vi "UpdateWeightsOutputLayer.vi"(0 "OutputH2":sgl[](array[numeric])=[0.0, 0.0], 1 "Final Output":sgl, 3 "dEtot_dOut":sgl, 4 "Learning Rate":sgl) -> ()   [LabVIEW 2020]
uses:
  <vilib>/rvi/Emulation/niFpgaSctlEmulationGetInTimedLoop.vi
  Global var FPGA.vi
  <vilib>/rvi/Memory/Memory_Emulation/nirvimemoryFastEmulation.vi
  <vilib>/rvi/Memory/Memory_Emulation/nirvimemoryEmulation.vi
  <vilib>/rvi/Emulation/niFpgaEmulationIsFPGAContextNoSignature.vi
  <vilib>/rvi/DataTransferAndStorage/Container/Common/niFpgaContainerGetUniqueNameForEmu.vi
  <vilib>/rvi/Emulation/niFpgaProcessEmulError.vi
  <vilib>/rvi/errors/nirviReportUnexpectedCaseInternalError (U32).vi
  <vilib>/rvi/DataTransferAndStorage/Container/XNode/niFpgaContainer.xnode
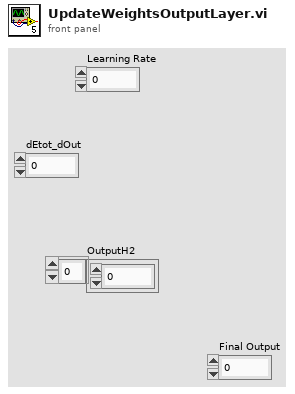
[diagram p1: front panel]
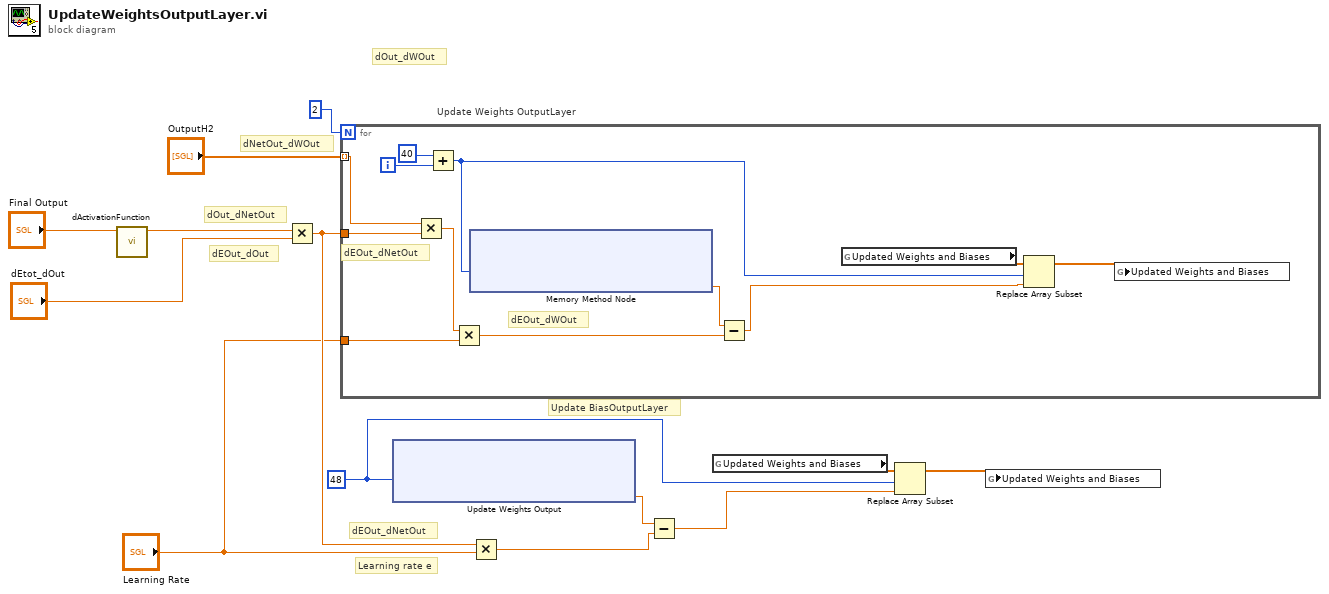
[diagram p0: block diagram]
diagram:
  w3 = u32 48 ("Address")
  # "Learning rate e"
  # "dEOut_dNetOut"
  # "dOut_dWOut"
  # "dEOut_dOut"
  # "Update BiasOutputLayer"
  # "dNetOut_dWOut"
  # "dOut_dNetOut"
  n1 = call "dActivationFunction.vi"("Output"="Final Output") -> ("f"=w8:sgl)  [unwired: 10 in]
  n2 = Multiply(x=w8, y="dEtot_dOut") -> (x*y=w6:sgl)
  n3 = for "Update Weights OutputLayer" {
    N: 2 -> [_]
    tunnel: "OutputH2" -> [w25] mode=indexing
    tunnel: w6 -> [w24]
    tunnel: "Learning Rate" -> [w19]
    i -> [w22]
    # "dEOut_dNetOut"
    # "dEOut_dWOut"
    n4 = Multiply(x=w25, y=w24) -> (x*y=w20:sgl)
    n5 = Add(x=i16 40, y=w22) -> (x+y=w14:i32)
    n6 = Multiply(x=w20, y=w19) -> (x*y=w18:sgl)
    n7 = xnode ("Memory Method Node")("Address"=w14) -> ("Data"=w21:sgl)  [unwired: 1 in, 1 out]
    n8 = Subtract(x=w21, y=w18) -> (x-y=w15:sgl)
    n9 = global read "Global var FPGA.vi" "Updated Weights and Biases"() -> (w17:sgl[])
    n10 = Replace Array Subset(array=w17, new element=w15, index=w14) -> (w16:sgl[])
    n11 = global write "Global var FPGA.vi" "Updated Weights and Biases"(w16) -> ()
  }
  n12 = xnode ("Update Weights Output")("Address"=w3) -> ("Data"=w10:sgl)  [unwired: 1 in, 1 out]
  n13 = Multiply(x=w6, y="Learning Rate") -> (x*y=w11:sgl)
  n14 = Subtract(x=w10, y=w11) -> (x-y=w1:sgl)
  n15 = global read "Global var FPGA.vi" "Updated Weights and Biases"() -> (w4:sgl[])
  n16 = Replace Array Subset(array=w4, new element=w1, index=w3) -> (w2:sgl[])
  n17 = global write "Global var FPGA.vi" "Updated Weights and Biases"(w2) -> ()
